vi "GetToken.vi"() -> (0 "error out":errorcluster, 1 "value":string)   [LabVIEW 2020]
uses:
  <vilib>/httpClient/POSTBuffer.vi
  <vilib>/httpClient/LabVIEWHTTPClient.lvlib
panel:
  out "body":string
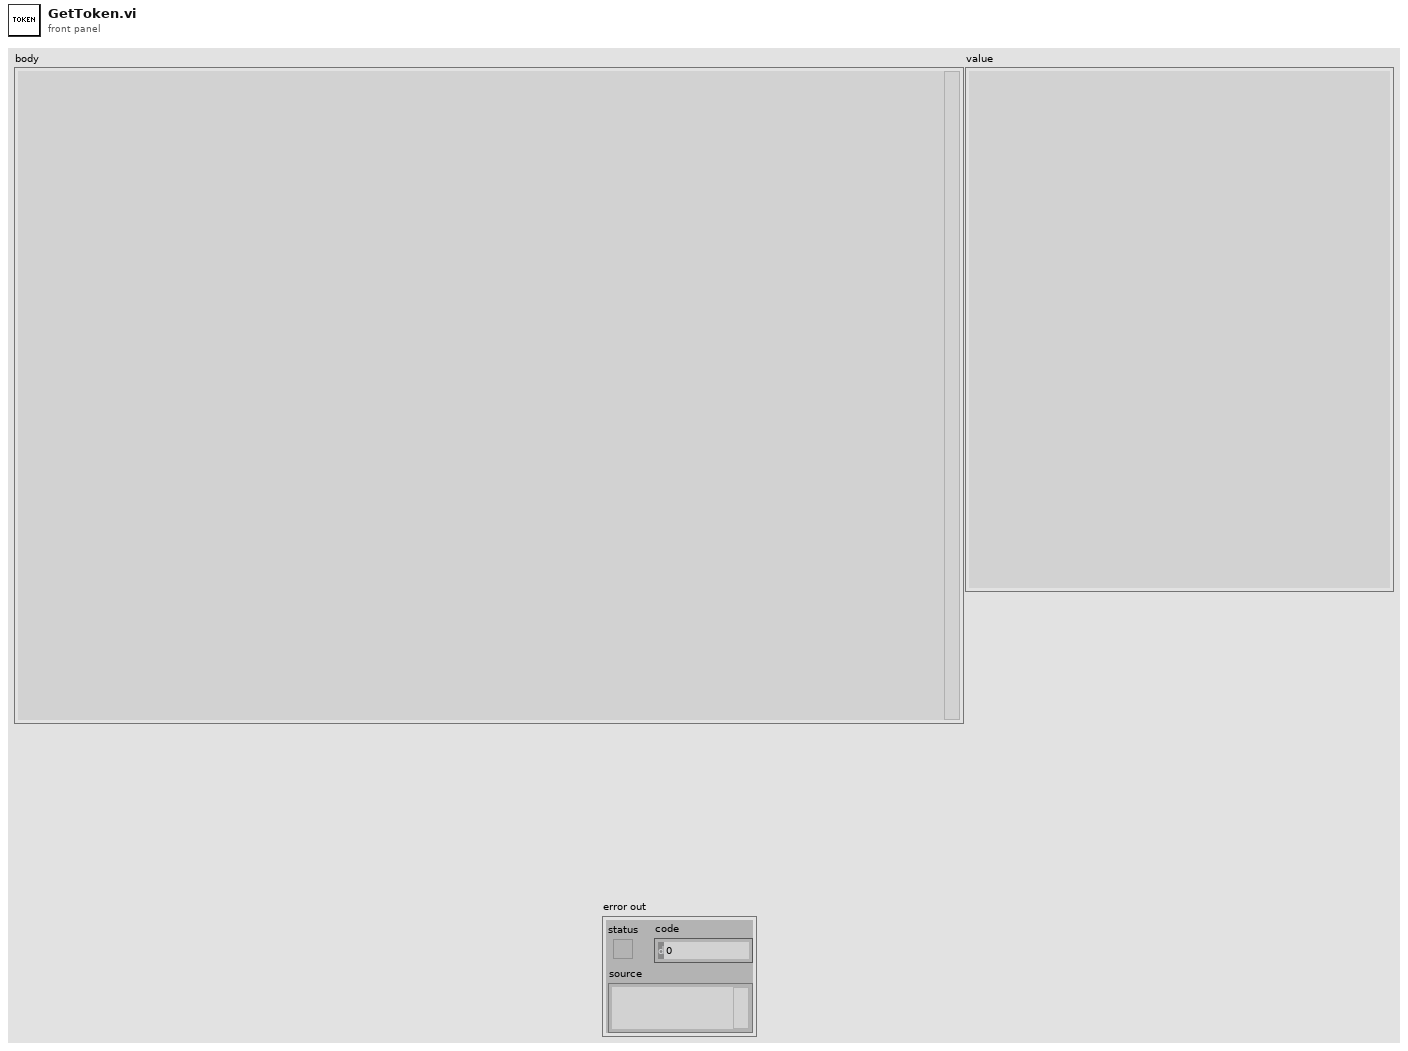
[diagram p1: front panel]
types:
  T1 = typedef "LabVIEWHTTPClient.lvlib/ClientHandle.ctl" = refnum<k1>
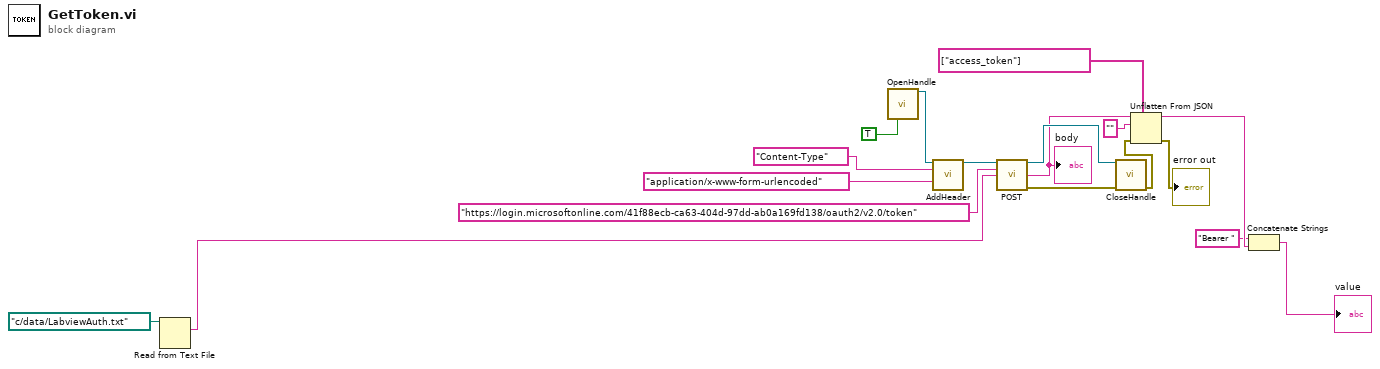
[diagram p0: block diagram]
diagram:
  n1 = Read from Text File(file (use dialog)=path "c:/data/LabviewAuth.txt") -> (text=w7:string)  [unwired: 3 in, 3 out]
  n2 = call <vilib>:"OpenHandle.vi"("verify server(true)"=TRUE) -> ("client handle out"=w12:T1)  [unwired: 13 in, 1 out]
  n3 = call <vilib>:"AddHeader.vi"("client handle"=w12, "header"="Content-Type", "value"="application/x-www-form-urlencoded") -> ("client handle out"=w13:T1)  [unwired: 11 in, 1 out]
  n4 = call-poly <vilib>:"POST.vi"("client handle"=w13, "url"="https://login.microsoftonline.com/41f88ecb-ca63-404d-97dd-ab0a169fd138/oauth2/v2.0/token", "buffer"=w7) -> ("client handle out"=w18:T1, "body"=w10:string, "error out"=w17:errorcluster)  [unwired: 9 in, 1 out]
  "body" <- w10
  n5 = call <vilib>:"CloseHandle.vi"("client handle"=w18, "error in (no error)"=w17) -> ("error out"=w5:errorcluster)  [unwired: 13 in]
  n6 = Unflatten From JSON(path=string[] ["access_token"], JSON string=w10, type and defaults="", error in (no error)=w5) -> (value=w3:string, error out=→"error out":errorcluster)  [unwired: 3 in]
  n7 = Concatenate Strings("Bearer " ("string"), w3) -> (→"value":string)
